vi "test_refnumLibrary.vi"(8 "error in (no error)":errorcluster) -> (0 "error out":errorcluster)   [LabVIEW 2013]
uses:
  run-tests/Run Test (LibraryRefnum).vi
  Caraya.lvlib
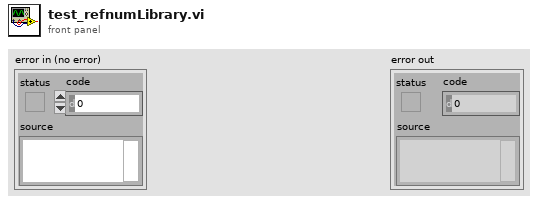
[diagram p1: front panel]
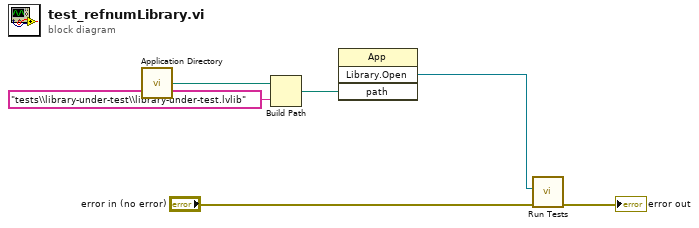
[diagram p0: block diagram]
diagram:
  n1 = call <vilib>:"Application Directory.vi"() -> ("Application Directory"=w4:path)
  n2 = Build Path(base path=w4, name or relative path="tests\\library-under-test\\library-under-test.lvlib") -> (appended path=w2:path)
  n3 = invoke class="App" method="Library.Open"("path"=w2) -> ("Open Library"=w1:refnum<vi>)  [unwired: 3 in, 3 out]
  n4 = call-poly "Run Tests.vi"("error in"="error in (no error)", "Library Refnum"=w1) -> ("error out"=→"error out":errorcluster)  [unwired: 9 in]
